vi "debounce button press and latch.vi"(11 "Boolean":bool) -> (3 "Boolean 2":bool=TRUE)   [LabVIEW 2014]
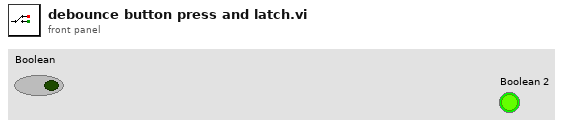
[diagram p1: front panel]
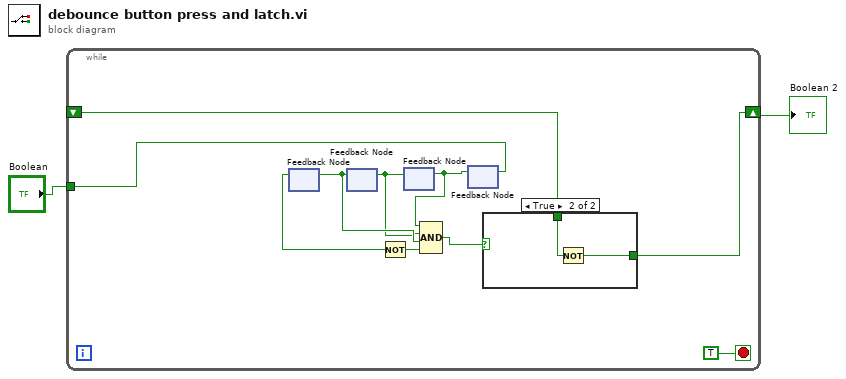
[diagram p0: block diagram]
diagram:
  n1 = while {
    shift-right: [w5] -> w2
    shift-left: _ -> [w4]
    tunnel: "Boolean" -> [w3]
    stop <- TRUE stop-if-true
    n2 = feedback #1() -> (w11:bool)  [unwired: 1 in]
    n3 = feedback #2() -> (w10:bool)  [unwired: 1 in]
    n4 = feedback-in #1(w10) -> ()
    n5 = Not(x=w11) -> (.not. x?=w12:bool)
    n6 = feedback #3() -> (w9:bool)  [unwired: 1 in]
    n7 = feedback-in #2(w9) -> ()
    n8 = feedback #4() -> (w8:bool)  [unwired: 1 in]
    n9 = feedback-in #3(w8) -> ()
    n10 = Compound Arithmetic op=AND(w8, w9, w10, w12) -> (w7:bool)
    n11 = feedback-in #4(w3) -> ()
    n12 = case shown="True" w7 {
      tunnel: [w13 w15] -> w5
      tunnel: w4 -> [w13 w14]
      frame False {
      }
      frame True {
        n13 = Not(x=w14) -> (.not. x?=w15:bool)
      }
    }
  }
  "Boolean 2" <- w2
